vi "CopyOutExample.vi"() -> ()   [LabVIEW 2019, in "libpqutility.lvlib"]
uses:
  libpqutility.lvlib
panel:
  in  "conninfo 2":T1={"host"="localhost", "port"="5432", "client_encoding"="WIN1251", "dbname"="data", "user"="postgres", "password"=""}
  in  "execute":bool
  in  "Stopp":bool
  in  "Command":string
  out "DatabaseMessages":T2={"PQerrorMessage"="", "PQStatus"=enum."CONNECTION_NEEDED", "PQresultErrorMessage"="", "PQresultStatus"=enum."PGRES_EMPTY_QUERY"}
  out "data":string[][](table)
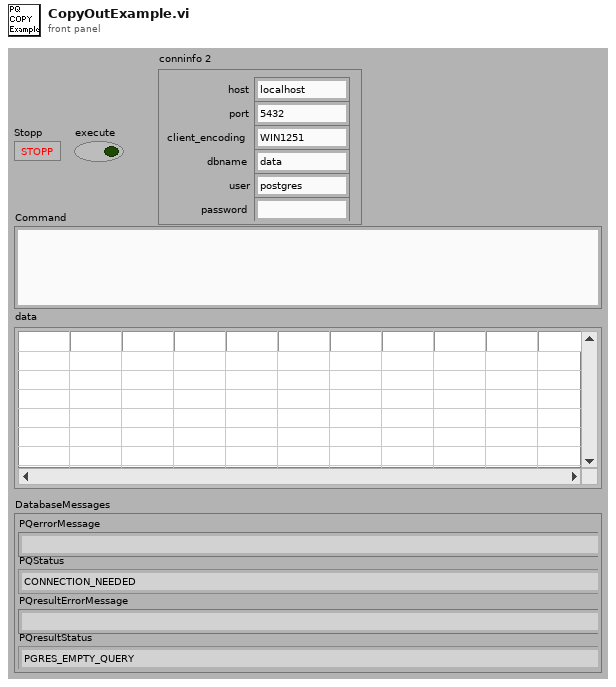
[diagram p1: front panel]
types:
  T1 = cluster{"host":string, "port":string, "client_encoding":string, "dbname":string, "user":string, "password":string}
  T2 = cluster{"PQerrorMessage":string, "PQStatus":enum16{"CONNECTION_OK", "CONNECTION_BAD", "CONNECTION_STARTED", "CONNECTION_MADE", "CONNECTION_AWAITING_RESPONSE", "CONNECTION_AUTH_OK", "CONNECTION_SETENV", "CONNECTION_SSL_STARTUP", "CONNECTION_NEEDED"}, "PQresultErrorMessage":string, "PQresultStatus":enum16{"PGRES_EMPTY_QUERY", "PGRES_COMMAND_OK", "PGRES_TUPLES_OK", "PGRES_COPY_OUT", "PGRES_COPY_IN", "PGRES_BAD_RESPONSE", "PGRES_NONFATAL_ERROR", "PGRES_FATAL_ERROR"}}
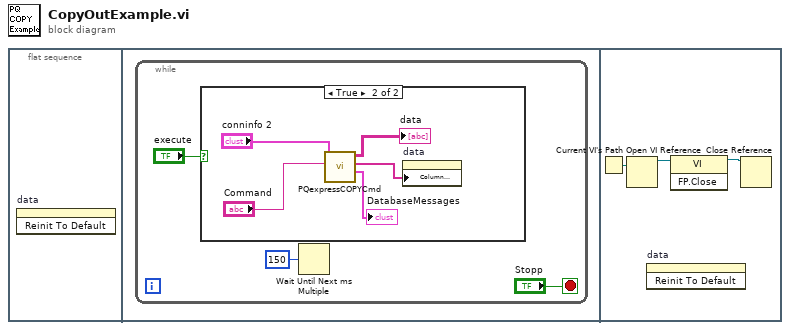
[diagram p0: block diagram]
diagram:
  n1 = flat-sequence {
    frame #0 {
      n2 = invoke on="data" class="Tbl (strikt)" method="Reinit To Default"() -> ()  [unwired: 3 in, 3 out]
    }
    frame #1 {
      n3 = while {
        stop <- "Stopp" stop-if-true
        n4 = case shown="True" "execute" {
          frame False {
          }
          frame True {
            n5 = call "PQexpressCOPYCmd.vi"("Command"="Command", "conninfo"="conninfo 2") -> ("DatabaseMessages"=→"DatabaseMessages":T2, "column_names"=w6:string[], "data"=→"data":string[][])  [unwired: 6 in, 1 out]
            n6 = property on="data" class="Tbl (strict)"("Column Headers[]"=w6) -> ()  [unwired: 2 in, 2 out]
          }
        }
        n7 = Wait Until Next ms Multiple ("Bis zum nächsten Vielfachen von ms warten")(millisecond multiple=u32 150 ("Vielfache von ms")) -> ()  [unwired: 1 out]
      }
    }
    frame #2 {
      n8 = Current VI's Path() -> (path=w11:path)
      n9 = Open VI Reference(vi path=w11) -> (vi reference=w10:refnum<vi>)  [unwired: 5 in, 1 out]
      n10 = invoke on="data" class="Tbl (strikt)" method="Reinit To Default"() -> ()  [unwired: 3 in, 3 out]
      n11 = invoke class="VI" method="FP.Close"(reference=w10) -> (reference out=w9:refnum<vi>)  [unwired: 2 in, 2 out]
      n12 = Close Reference(reference=w9) -> ()  [unwired: 1 in, 1 out]
    }
  }
